vi "Open.vi"(8 "error in (no error)":errorcluster, 11 "DeploySerialResource in":refnum<class "SerialResource.lvclass">) -> (0 "error out":errorcluster, 3 "DeploySerialResource out":refnum<class "SerialResource.lvclass">)   [LabVIEW 2020]
uses:
  SerialResource.lvclass/SerialResource.ctl
  SerialResource.lvclass
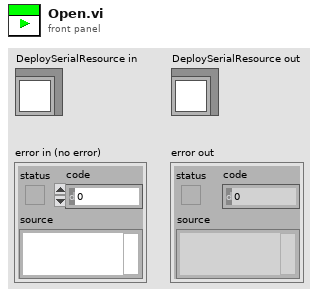
[diagram p1: front panel]
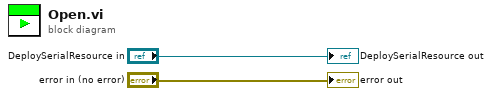
[diagram p0: block diagram]
diagram:
  "error out" <- "error in (no error)"
  "DeploySerialResource out" <- "DeploySerialResource in"
